vi "3.1.1-VectorNav Read.vi"(10 "error in":errorcluster, 11 "FPGA Ref In":T1) -> (1 "Final Reply":string, 2 "error out":errorcluster, 3 "FPGA VI Reference Out":T1)   [LabVIEW 2010]
doc: "This VI reads data out of the Read FIFO. It converts the individual bytes to a string and does some primitive parsing and error handling."
uses:
  2-Low Neurons/2-FPGA VI Typedef.ctl
  3.1.1-VectorNav Parser.ctl
  <vilib>/rvi/interface/nirviMethod/nirviMethod.xnode
  FPGA Bitfiles/DaveBrain_FPGATarget_1-Hindbrain_F0E489D8.lvbitx
  1-Hindbrain.vi
  <vilib>/rvi/interface/common/niFpgaNodeNameForErrorReporting.ctl
  <vilib>/rvi/errors/niLvFpgaWhatHappensToTopLevelVI.ctl
  <vilib>/Utility/error.llb/Error Cluster From Error Code.vi
  3.0-Global.vi
  <vilib>/rvi/errors/niLvFpgaAdjustHostInterfaceError.vi
  NiFpgaLv.dll
panel:
  out "Data":string
  out "Elements Remaining":u32
  out "Checksum":string
  out "String":string
  in  "stop":bool
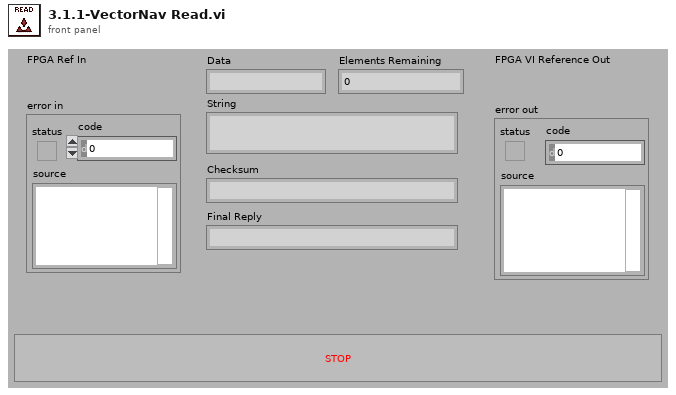
[diagram p1: front panel]
types:
  T1 = typedef "2-FPGA VI Typedef.ctl" = refnum<k20>
  T2 = typedef "3.1.1-VectorNav Parser.ctl" = enum16{"Wait for $", "Read values", "Checksum", "Error", "Done"}
  T3 = typedef "niFpgaNodeNameForErrorReporting.ctl" = enum16{"Open FPGA VI Reference", "Read/Write Control", "Invoke Method: Abort", "Invoke Method: Acknowledge IRQ", "Invoke Method: Download", "Invoke Method: FIFO.Configure", "Invoke Method: FIFO.Read", "Invoke Method: FIFO.Start", "Invoke Method: FIFO.Stop", "Invoke Method: FIFO.Write", "Invoke Method: Reset", "Invoke Method: Run", "Invoke Method: Wait on IRQ", "Close FPGA VI Reference"}
  T4 = typedef "niLvFpgaWhatHappensToTopLevelVI.ctl" = enum16{"top level VI scripted behind XNode", "top level VI inlined behind XNode"}
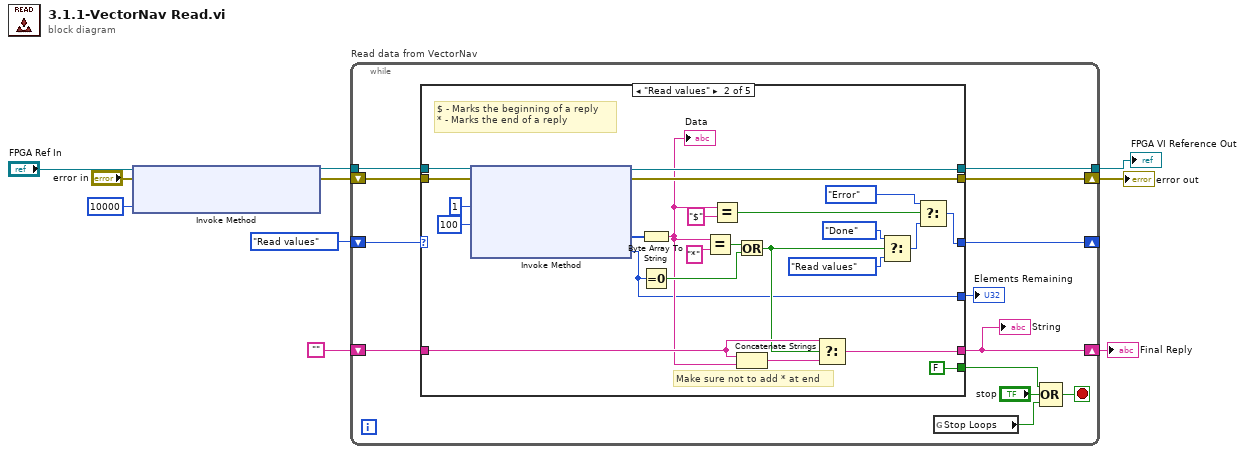
[diagram p0: block diagram]
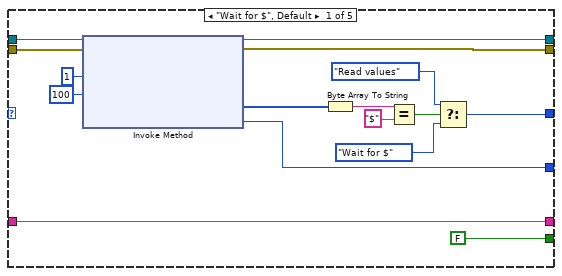
[diagram p2: hidden frame]
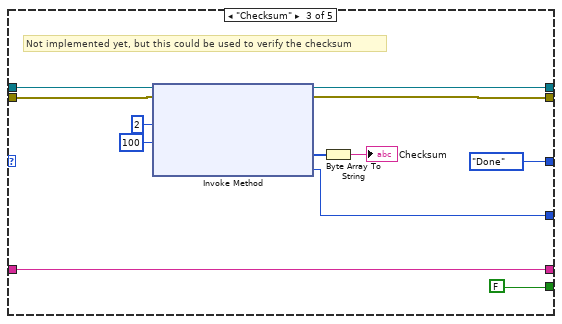
[diagram p3: hidden frame]
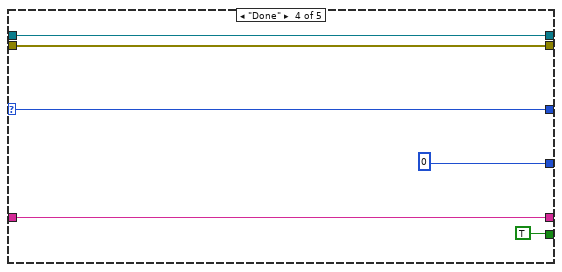
[diagram p4: hidden frame]
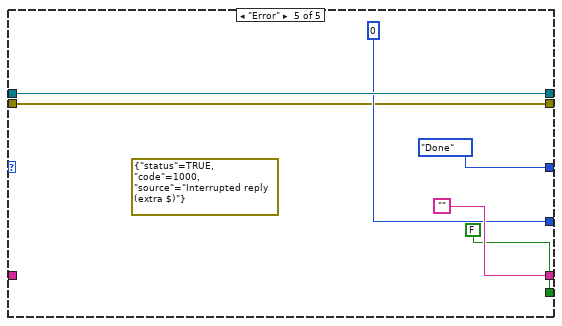
[diagram p5: hidden frame]
diagram:
  n1 = xnode "Invoke Method"("FPGA VI Reference In"="FPGA Ref In", "error in"="error in", "Depth"=u32 10000) -> ("FPGA VI Reference Out"=w5:T1, "error out"=w9:errorcluster)
  n2 = while "Read data from VectorNav" {
    shift-right: [w15] -> w6
    shift-left: "" -> [w19]
    shift-right: [w21] -> _
    shift-left: 3.1.1-VectorNav_Parser."Read values" ("Enum") -> [w20]
    shift-right: [w12] -> w4
    shift-left: w9 -> [w17]
    tunnel: w5 -> [w14]
    tunnel: [w13] -> w1
    stop <- w22 stop-if-true
    n3 = case shown="\"Read values\"" w20 {
      selector: w20 -> [_ _ _ w293 _]
      tunnel: [w31 w118 3.1.1-VectorNav_Parser."Done" ("Enum") w293 3.1.1-VectorNav_Parser."Done" ("Enum")] -> w21
      tunnel: w19 -> [w30 w128 w214 w297 _]
      tunnel: [w30 w127 w214 w297 ""] -> w15
      tunnel: [FALSE FALSE FALSE TRUE FALSE] -> w18
      tunnel: w14 -> [w28 w125 w212 w295 w303]
      tunnel: w17 -> [w27 w124 w211 w294 w298]
      tunnel: [w26 w123 w210 w295 w303] -> w13
      tunnel: [w25 w122 w209 w294 w298] -> w12
      tunnel: [w24 w112 w208 u32 0 ("Elements Remaining") u32 0 ("Elements Remaining")] -> w16
      frame "Wait for $", Default {
        n4 = xnode "Invoke Method"("FPGA VI Reference In"=w28, "error in"=w27, "Number of Elements"=u32 1, "Timeout (ms)"=100) -> ("FPGA VI Reference Out"=w26:T1, "error out"=w25:errorcluster, "Data"=w39:u8[], "Elements Remaining"=w24:u32)
        n5 = Byte Array To String(unsigned byte array=w39) -> (string=w34:string)
        n6 = Equal?(x=w34, y="$") -> (x = y?=w35:bool)
        n7 = Select(t=3.1.1-VectorNav_Parser."Read values" ("Enum"), s=w35, f=3.1.1-VectorNav_Parser."Wait for $" ("Enum")) -> (s? t:f=w31:T2)
      }
      frame "Read values" {
        # "Make sure not to add * at end"
        # "$ - Marks the beginning of a reply\n* - Marks the end of a reply"
        n8 = xnode "Invoke Method"("FPGA VI Reference In"=w125, "error in"=w124, "Number of Elements"=u32 1, "Timeout (ms)"=100) -> ("FPGA VI Reference Out"=w123:T1, "error out"=w122:errorcluster, "Data"=w130:u8[], "Elements Remaining"=w112:u32)
        n9 = Byte Array To String(unsigned byte array=w130) -> (string=w113:string)
        "Data" <- w113
        n10 = Equal To 0?(x=w112) -> (x = 0?=w117:bool)
        n11 = Equal?(x=w113, y="*") -> (x = y?=w116:bool)
        n12 = Equal?(x=w113, y="$") -> (x = y?=w114:bool)
        n13 = Or(x=w116, y=w117) -> (x .or. y?=w115:bool)
        n14 = Concatenate Strings(w128, w113) -> (w129:string)
        n15 = Select(t=w128, s=w115, f=w129) -> (s? t:f=w127:string)
        n16 = Select(t=3.1.1-VectorNav_Parser."Done" ("Enum"), s=w115, f=3.1.1-VectorNav_Parser."Read values" ("Enum")) -> (s? t:f=w119:T2)
        n17 = Select(t=3.1.1-VectorNav_Parser."Error" ("Enum"), s=w114, f=w119) -> (s? t:f=w118:T2)
      }
      frame "Checksum" {
        # "Not implemented yet, but this could be used to verify the checksum"
        n18 = xnode "Invoke Method"("FPGA VI Reference In"=w212, "error in"=w211, "Number of Elements"=u32 2, "Timeout (ms)"=100) -> ("FPGA VI Reference Out"=w210:T1, "error out"=w209:errorcluster, "Data"=w217:u8[], "Elements Remaining"=w208:u32)
        n19 = Byte Array To String(unsigned byte array=w217) -> (string=→"Checksum":string)
      }
      frame "Done" {
      }
      frame "Error" {
        (unwired) errorcluster {"status"=TRUE, "code"=1000, "source"="Interrupted reply (extra $)"} ("error in")
      }
    }
    "Elements Remaining" <- w16
    "String" <- w15
    n20 = global read "3.0-Global.vi" "Stop Loops"() -> (w11:bool)
    n21 = Compound Arithmetic op=OR(w18, "stop", w11) -> (w22:bool)
  }
  "Final Reply" <- w6
  "error out" <- w4
  "FPGA VI Reference Out" <- w1
